vi "Show Errors.vi"(8 "error in (no error)":errorcluster, 10 "Node In (localnode.)":string="localnode.", 11 "VISA resource name":refnum<visa-resource-name>) -> (0 "error out":errorcluster, 2 "Node Out":string="localnode.", 3 "VISA resource name out":refnum<visa-resource-name>, 4 "Command String":string)   [LabVIEW 2012, in "Keithley 2600 Series.lvlib"]
doc: "Enables/Disables the automatic showing of errors.\n\nWhen enabled, errors are sent the to the output data queue immediately after they occur.\n\n<b>Functions and Attributes Used</b>\nlocalnode.showerrors"
uses:
  Keithley 2600 Series.lvlib
panel:
  in  "Show Errors (Off)":bool
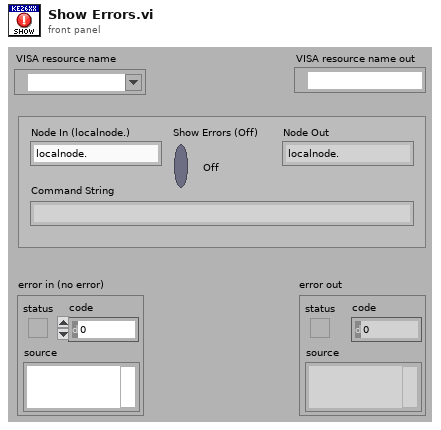
[diagram p1: front panel]
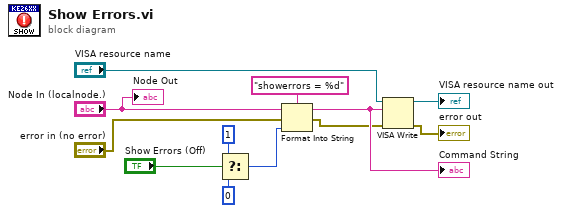
[diagram p0: block diagram]
diagram:
  n1 = Select(t=1, s="Show Errors (Off)", f=0) -> (s? t:f=w3:i32)
  n2 = Format Into String(format string="showerrors = %d", initial string="Node In (localnode.)", error in="error in (no error)", w3) -> (resulting string=w2:string, error out=w1:errorcluster)
  "Command String" <- w2
  n3 = VISA Write(VISA resource name="VISA resource name", write buffer=w2, error in (no error)=w1) -> (VISA resource name out=→"VISA resource name out":refnum<visa-resource-name>, error out=→"error out":errorcluster)  [unwired: 1 out]
  "Node Out" <- "Node In (localnode.)"
